vi "GEOM_GetRoi2Str.vi"() -> (2 "roi":string, 4 "ysize":u32, 5 "xsize":u32, 6 "ystart":u32, 7 "xstart":u32)   [LabVIEW 2016]
uses:
  GEOM_VAR_action.ctl
  GEOM_Gbls.vi
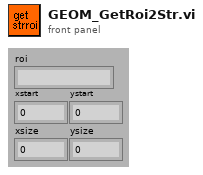
[diagram p1: front panel]
types:
  T1 = typedef "GEOM_VAR_action.ctl" = enum16{"read", "write"}
  T2 = typedef "GEOM_Coords.ctl" = cluster{"xstart":u32, "ystart":u32, "xsize":u32, "ysize":u32}
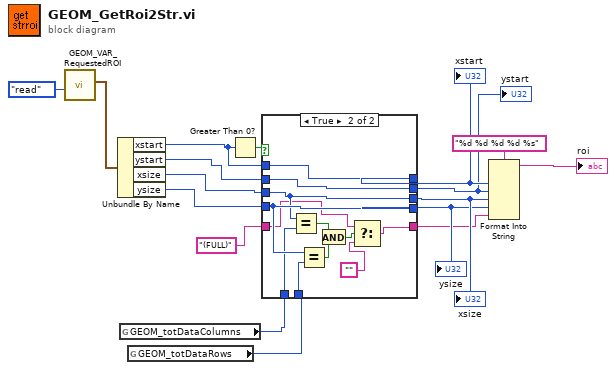
[diagram p0: block diagram]
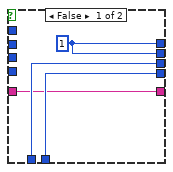
[diagram p2: hidden frame]
diagram:
  n1 = call "GEOM_VAR_RequestedROI.vi"("Action"=GEOM_VAR_action."read") -> ("GEOM_RequestedROI out"=w3:T2)  [unwired: 1 in, 9 out]
  n2 = Unbundle By Name(w3) -> ("xstart"=w15:u32, "ystart"=w13:u32, "xsize"=w11:u32, "ysize"=w9:u32)
  n3 = global read "GEOM_Gbls.vi" "GEOM_totDataColumns"() -> (w7:u16)
  n4 = global read "GEOM_Gbls.vi" "GEOM_totDataRows"() -> (w6:u16)
  n5 = Greater Than 0?(x=w15) -> (x > 0?=w16:bool)
  n6 = case shown="True" w16 {
    tunnel: w15 -> [_ w33]
    tunnel: [w21 w33] -> w14
    tunnel: w13 -> [_ w32]
    tunnel: [w21 w32] -> w12
    tunnel: w11 -> [_ w25]
    tunnel: [w20 w25] -> w10
    tunnel: w9 -> [_ w27]
    tunnel: [w19 w27] -> w8
    tunnel: w7 -> [w20 w26]
    tunnel: w6 -> [w19 w28]
    tunnel: [w18 w23] -> w5
    tunnel: "(FULL)" -> [w18 w24]
    frame False {
      w21 = u32 1 ("xstart")
    }
    frame True {
      n7 = Equal?(x=w25, y=w26) -> (x = y?=w31:bool)
      n8 = Equal?(x=w27, y=w28) -> (x = y?=w30:bool)
      n9 = And(x=w31, y=w30) -> (x .and. y?=w29:bool)
      n10 = Select(t=w24, s=w29, f="") -> (s? t:f=w23:string)
    }
  }
  "xstart" <- w14
  "ystart" <- w12
  "xsize" <- w10
  "ysize" <- w8
  n11 = Format Into String(format string="%d %d %d %d %s", w14, w12, w10, w8, w5) -> (resulting string=→"roi":string)  [unwired: 2 in, 1 out]
